vi "Main.vi"() -> ()   [LabVIEW 2018]
doc: "The myRIO Project template acquires acceleration data from the onboard accelerometer and displays the changes of acceleration values in a waveform chart."
uses:
  <vilib>/myRIO/Instrument Drivers/Utilities/Utilities.lvlib
  <vilib>/imath/engines/lvmath2/RunTimeEngine/Managers/WorkSpace/UID Generator.vi
  <vilib>/imath/engines/lvmath/Plug In/_Char/NIMS_CH_String to Character Array.vi
  <vilib>/imath/engines/lvmath/Plug In/_Char/NIMS_CH_character datatype.ctl
  <vilib>/imath/engines/lvmath2/RunTimeEngine/IndexRead/NIMS V(S).vi
  <vilib>/imathl/engines/lvmath/Functions/Error Handling/Create Error.vi
  <vilib>/imath/engines/lvmath2/RunTimeEngine/LocalVariableDefStatement/MC_LocalVariableDefStatement_Display.vi
  <vilib>/imath/engines/lvmath2/RunTimeEngine/RunTimeType/NIMS_RunTimeType_From StrictType (excl LVString).vi
  <vilib>/imath/engines/lvmath2/RunTimeEngine/Managers/SymbolTable/Clear UID.vi
  <vilib>/imath/engines/lvmath2/RunTimeEngine/Managers/SymbolTable/NIMS_WorkSpace.lvlib
  <vilib>/imath/engines/lvmath2/RunTimeEngine/NodeEndStatement/NIMS_NodeEndStatement_Output.vi
  <vilib>/imath/engines/lvmath2/RunTimeEngine/ErrorHandling/NIMS_Finalize Error.vi
  <vilib>/Analysis/NI_AALPro.lvlib
  <vilib>/imath/engines/lvmath2/RunTimeEngine/IndexReplace/NIMS M(S,S)=S.vi
  <vilib>/imath/engines/lvmath2/RunTimeEngine/ErrorHandling/NIMS_Create Error From Enums.vi
  <vilib>/imath/engines/lvmath2/RunTimeEngine/RangeToken/NIMS_Range_R2 - Integer.vi
  <vilib>/imath/engines/lvmath2/RunTimeEngine/CommandStatement/MC_CommandStatement_break.vi
  <vilib>/imath/engines/lvmath2/RunTimeEngine/IndexRead/NIMS M(S,S).vi
  <vilib>/robotics/Navigation/shared/WorldMap/OccupancyGridWorldMap/NI_Robotics_OccupancyGridWorldMap.lvclass
  <vilib>/imath/engines/lvmath2/RunTimeEngine/BuiltInFunctions/acos/NIMS_acos(C).vi
  <vilib>/Analysis/coordinate.llb/2D Cartesian Coordinate Rotation (Scalar).vi
  <vilib>/robotics/Navigation/shared/MapNode/OccupancyGridNode/NI_Robotics_OccupancyGridMapNode.lvclass
  C:/Program Files (x86)/National Instruments/LabVIEW 2018/vi.lib/robotics/Navigation/shared/MapNode/AbstractAstarNode/NI_Robotics_AbstractAstarNode.lvclass
  <vilib>/imath/engines/lvmath2/RunTimeEngine/BuiltInFunctions/round/NIMS_round(DBL-S).vi
  <vilib>/imath/engines/lvmath2/RunTimeEngine/BuiltInFunctions/char/NIMS_char.vi
  <vilib>/imath/engines/lvmath/Plug In/_Char/NIMS_CH_String CV to Character 2D.vi
  <vilib>/imath/engines/lvmath2/RunTimeSupport/NIMS_Error if Not Equal.vi
  <vilib>/imath/engines/lvmath2/RunTimeEngine/BuiltInFunctions/min/2 inputs/NIMS_min(RG,RG)-no size check.vi
  <vilib>/imath/engines/lvmath2/RunTimeEngine/BuiltInFunctions/max/2 inputs/NIMS_max(RG,RG)-no size check.vi
  <vilib>/imath/engines/lvmath/Plug In/_Char/NIMS_CH_Character 2D to String 1D.vi
  <vilib>/imath/engines/lvmath2/RunTimeEngine/BuiltInFunctions/mod/NIMS_mod_no_size_check.vi
  <vilib>/imath/engines/lvmath2/RunTimeEngine/VariableToken/NIMS_VariableToken_CondDefined.vi
  <vilib>/imath/engines/lvmath/Functions/Error Handling/MergeErrorsWrapper.vi
panel:
  out "field":i32[][](array[numeric])
  out "error out":errorcluster
  in  "stop":bool
  in  "Tab Control":enum32{"Main", "Settings"}(tab)
  out "Dist Finish":dbl
  out "Theta Finish":dbl
  out "Read Camera":bool
  out "Data":string
  out "Position":cluster{"X":dbl, "Y":dbl, "Theta":dbl}
  out "X Finish":string[](array[string])
  out "Y Finish":string[](array[string])
  out "G":i32[][](array[numeric])
  in  "Motor Controller ID#  (I2C Address)":u8=1 min=1 max=4
  in  "Motor Controller ID#  (I2C Address) 2":u8=2 min=1 max=4
  in  "Servo Controller ID#  (I2C Address) 3":u8=3 min=1 max=4
  in  "Controller myRIO MXP Port A/B":tag="A/I2C"
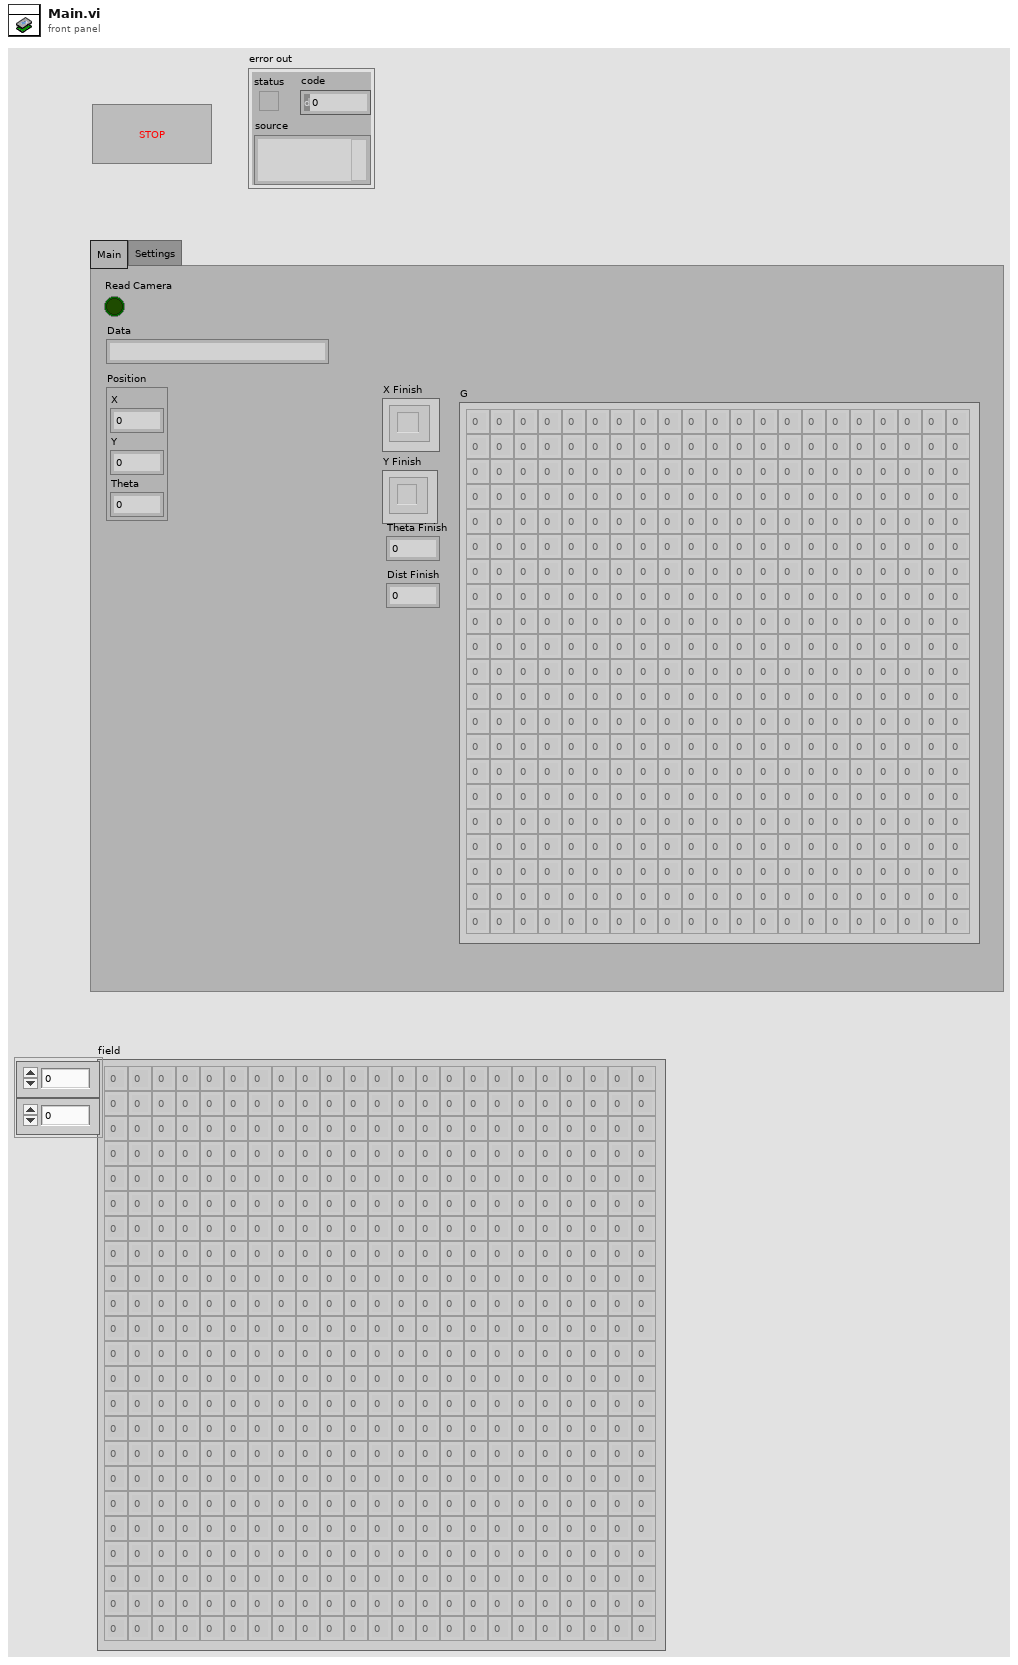
[diagram p1: front panel]
types:
  T1 = typedef "NIMS_CH_character datatype.ctl" = cluster{"Numeric":u8}
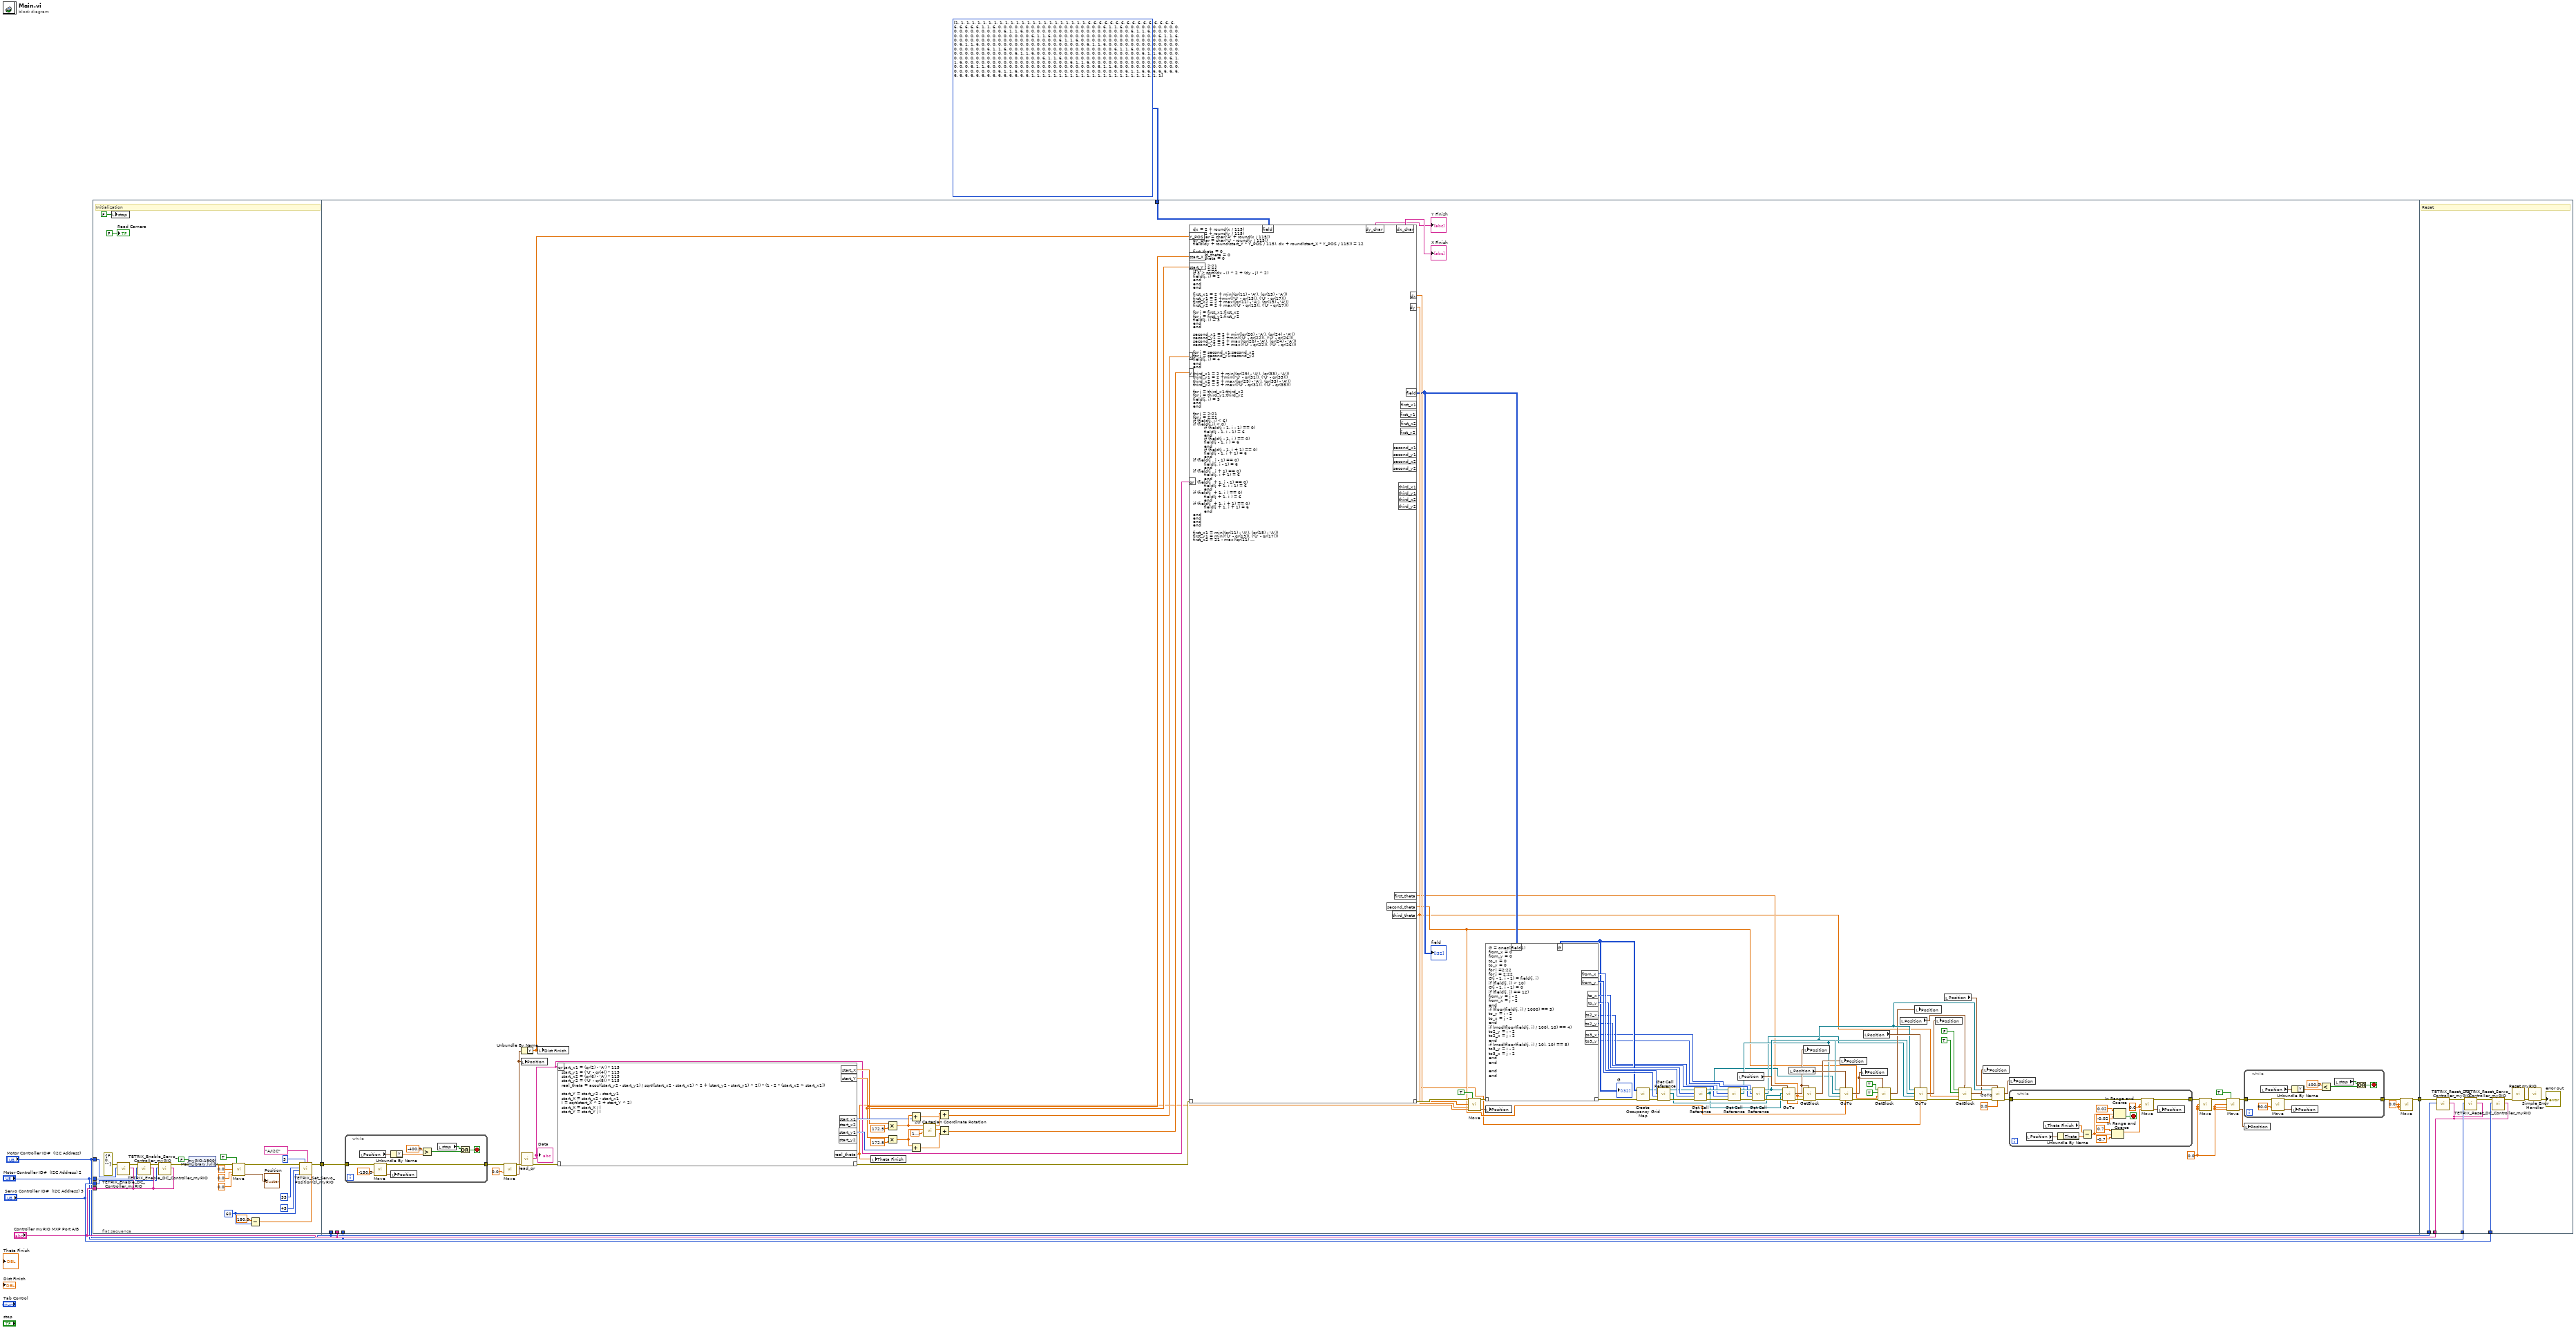
[diagram p0: block diagram]
diagram:
  n1 = flat-sequence {
    tunnel: "Motor Controller ID#  (I2C Address)" -> [w32]
    tunnel: "Motor Controller ID#  (I2C Address) 2" -> [w31]
    tunnel: "Controller myRIO MXP Port A/B" -> [w26]
    tunnel: "Servo Controller ID#  (I2C Address) 3" -> [w9]
    tunnel: [w10] -> w3
    tunnel: "Controller myRIO MXP Port A/B" -> [_]
    tunnel: "Motor Controller ID#  (I2C Address)" -> [_]
    tunnel: "Motor Controller ID#  (I2C Address) 2" -> [_]
    tunnel: w3 -> [w126]
    tunnel: u8[][] [[1, 1, 1, 1, 1, 1, 1, 1, 1, 1, 1, 1, 1, 1, 1, 1, 1, 1, 1, 1, 1, 1, 1], [1, 6, 6, 6, 6, 6, 6, 6, 6, 6, 6, 6, 6, 6, 6, 6, 6, 6, 6, 6, 6, 6, 1], [1, 6, 0, 0, 0, 0, 0, 0, 0, 0, 0, 0, 0, 0, 0, 0, 0, 0, 0, 0, 0, 6, 1], [1, 6, 0, 0, 0, 0, 0, 0, 0, 0, 0, 0, 0, 0, 0, 0, 0, 0, 0, 0, 0, 6, 1], [1, 6, 0, 0, 0, 0, 0, 0, 0, 0, 0, 0, 0, 0, 0, 0, 0, 0, 0, 0, 0, 6, 1], [1, 6, 0, 0, 0, 0, 0, 0, 0, 0, 0, 0, 0, 0, 0, 0, 0, 0, 0, 0, 0, 6, 1], [1, 6, 0, 0, 0, 0, 0, 0, 0, 0, 0, 0, 0, 0, 0, 0, 0, 0, 0, 0, 0, 6, 1], [1, 6, 0, 0, 0, 0, 0, 0, 0, 0, 0, 0, 0, 0, 0, 0, 0, 0, 0, 0, 0, 6, 1], [1, 6, 0, 0, 0, 0, 0, 0, 0, 0, 0, 0, 0, 0, 0, 0, 0, 0, 0, 0, 0, 6, 1], [1, 6, 0, 0, 0, 0, 0, 0, 0, 0, 0, 0, 0, 0, 0, 0, 0, 0, 0, 0, 0, 6, 1], [1, 6, 0, 0, 0, 0, 0, 0, 0, 0, 0, 0, 0, 0, 0, 0, 0, 0, 0, 0, 0, 6, 1], [1, 6, 0, 0, 0, 0, 0, 0, 0, 0, 0, 0, 0, 0, 0, 0, 0, 0, 0, 0, 0, 6, 1], [1, 6, 0, 0, 0, 0, 0, 0, 0, 0, 0, 0, 0, 0, 0, 0, 0, 0, 0, 0, 0, 6, 1], [1, 6, 0, 0, 0, 0, 0, 0, 0, 0, 0, 0, 0, 0, 0, 0, 0, 0, 0, 0, 0, 6, 1], [1, 6, 0, 0, 0, 0, 0, 0, 0, 0, 0, 0, 0, 0, 0, 0, 0, 0, 0, 0, 0, 6, 1], [1, 6, 0, 0, 0, 0, 0, 0, 0, 0, 0, 0, 0, 0, 0, 0, 0, 0, 0, 0, 0, 6, 1], [1, 6, 0, 0, 0, 0, 0, 0, 0, 0, 0, 0, 0, 0, 0, 0, 0, 0, 0, 0, 0, 6, 1], [1, 6, 0, 0, 0, 0, 0, 0, 0, 0, 0, 0, 0, 0, 0, 0, 0, 0, 0, 0, 0, 6, 1], [1, 6, 0, 0, 0, 0, 0, 0, 0, 0, 0, 0, 0, 0, 0, 0, 0, 0, 0, 0, 0, 6, 1], [1, 6, 0, 0, 0, 0, 0, 0, 0, 0, 0, 0, 0, 0, 0, 0, 0, 0, 0, 0, 0, 6, 1], [1, 6, 0, 0, 0, 0, 0, 0, 0, 0, 0, 0, 0, 0, 0, 0, 0, 0, 0, 0, 0, 6, 1], [1, 6, 6, 6, 6, 6, 6, 6, 6, 6, 6, 6, 6, 6, 6, 6, 6, 6, 6, 6, 6, 6, 1], [1, 1, 1, 1, 1, 1, 1, 1, 1, 1, 1, 1, 1, 1, 1, 1, 1, 1, 1, 1, 1, 1, 1]] ("Field") -> [w105]
    tunnel: [w59] -> w1
    tunnel: "Controller myRIO MXP Port A/B" -> [w4697]
    tunnel: "Motor Controller ID#  (I2C Address)" -> [w4701]
    tunnel: "Motor Controller ID#  (I2C Address) 2" -> [w4700]
    tunnel: "Servo Controller ID#  (I2C Address) 3" -> [w4698]
    tunnel: w1 -> [w4693]
    frame #0 {
      w16 = u8 60 ("Servo 4 Position (0 - 180 degrees)")
      # "Initialization"
      n2 = local write "stop"(FALSE ("Stop")) -> ()
      n3 = call <vilib>:"TETRIX_Enable_DC_Controller_myRIO.vi"("myRIO MXP Port A/B"=w26, "Controller ID#  (I2C Address)"=w32, "Error/Flow In"=errorcluster {"status"=FALSE, "code"=0, "source"=""}) -> ("Error/Flow Out"=w33:errorcluster)  [unwired: 4 in]
      n4 = call <vilib>:"TETRIX_Enable_DC_Controller_myRIO.vi"("myRIO MXP Port A/B"=w26, "Controller ID#  (I2C Address)"=w31, "Error/Flow In"=w33) -> ("Error/Flow Out"=w29:errorcluster)  [unwired: 4 in]
      n5 = call <vilib>:"TETRIX_Enable_Servo_Controller_myRIO.vi"("myRIO MXP Port A/B"=w26, "Controller ID#  (I2C Address)"=w9, "Error/Flow In"=w29) -> ("Error/Flow Out"=w28:errorcluster)  [unwired: 4 in]
      n6 = shared-variable "myRIO-1900\\MainLibrary.lvlib\\stop"(FALSE ("Stop"), error in=w28) -> (error out=w23:errorcluster)
      n7 = call "Move.vi"("Error/Flow In"=w23, "Reset"=TRUE, "x (mm/s)"=0.0, "y (mm/s)"=0.0, "theta (rad/s)"=0.0) -> ("Error/Flow Out"=w11:errorcluster, "Position"=→"Position":cluster{"X":dbl, "Y":dbl, "Theta":dbl})  [unwired: 9 in]
      n8 = Subtract(x=180.0, y=w16) -> (x-y=w15:dbl)
      n9 = call <vilib>:"TETRIX_Set_Servo_Position(s)_myRIO.vi"("Servo 4 Position (0 - 180 degrees)"=w15, "myRIO MXP Port A/B"=tag "A/I2C", "Controller ID#  (I2C Address)"=u8 3, "Servo 3 Position (0 - 180 degrees)"=w16, "Servo 2 Position (0 - 180 degrees)"=u8 45, "Servo 1 Position (0 - 180 degrees)"=u8 35 ("Controller ID#  (I2C Address)"), "Error/Flow In"=w11) -> ("Error/Flow Out"=w10:errorcluster)  [unwired: 2 in]
      "Read Camera" <- FALSE ("Read Camera")
    }
    frame #1 {
      w58 = 0.0 ("x (mm/s)")
      w63 = 0.0 ("x (mm/s)")
      n10 = while {
        tunnel: [w4688] -> w125
        tunnel: w126 -> [w4689]
        stop <- w4683 stop-if-true
        n11 = local read "Position"() -> (w4692:cluster{"X":dbl, "Y":dbl, "Theta":dbl})
        n12 = call "Move.vi"("Error/Flow In"=w4689, "y (mm/s)"=-150.0) -> ("Error/Flow Out"=w4688:errorcluster, "Position"=w4687:cluster{"X":dbl, "Y":dbl, "Theta":dbl})  [unwired: 12 in]
        n13 = Unbundle By Name(w4692) -> ("Y"=w4691:dbl)
        n14 = local write "Position"(w4687) -> ()
        n15 = Greater?(x=-400.0, y=w4691) -> (0:w4684:bool)
        n16 = local read "stop"() -> (w4685:bool)
        n17 = Or(x=w4685, y=w4684) -> (x .or. y?=w4683:bool)
      }
      n18 = call "Move.vi"("Error/Flow In"=w125, "y (mm/s)"=0.0) -> ("Error/Flow Out"=w127:errorcluster, "Position"=w106:cluster{"X":dbl, "Y":dbl, "Theta":dbl})  [unwired: 12 in]
      n19 = Unbundle By Name(w106) -> ("Y"=w89:dbl)
      n20 = local write "Position"(w106) -> ()
      n21 = call "read_qr.vi"("error in"=w127) -> ("error out"=w108:errorcluster, "Data"=w109:string)  [unwired: 8 in]
      "Data" <- w109
      n22 = local write "Dist Finish"(w89) -> ()
      n23 = mathscript code="start_x1 = (qr(2) - 'A') * 115\nstart_y1 = ('U' - qr(4)) * 115\nstart_x2 = (qr(6) - 'A') * 115\nstart_y2 = ('U' - qr(8)) * 115\nreal_theta = acos((start_y2 - start_y1) / sqrt((start_x2 - start_x1) ^ 2 + (start_y2 - start_y1) ^ 2)) * (1 - 2 * (start_x2 > start_x1))\n\nstart_Y = start_y2 - start_y1\nstart_X = start_x2 - start_x1\nl = sqrt(start_X ^ 2 + start_Y ^ 2)\nstart_X = start_X / l\nstart_Y = start_Y / l"("??"=w108, "qr"=w109) -> ("??"=w107:errorcluster, "real_theta"=w57:cdb, "start_x1"=w115:i32, "start_y1"=w114:i32, "start_X"=w113:dbl, "start_Y"=w112:dbl)  [unwired: 2 out]
      n24 = local write "Theta Finish"(w57) -> ()
      n25 = Multiply(x=w113, y=172.5) -> (x*y=w118:dbl)
      n26 = Multiply(x=w112, y=172.5) -> (x*y=w119:dbl)
      n27 = Add(x=w118, y=w115) -> (x+y=w120:dbl)
      n28 = Add(x=w119, y=w114) -> (x+y=w122:dbl)
      n29 = call-poly <vilib>:"2D Cartesian Coordinate Rotation.vi"("theta"=1.5707963267948966, "y"=w119, "x"=w118) -> ("y out"=w123:dbl, "x out"=w121:dbl)  [unwired: 6 in, 1 out]
      n30 = Add(x=w121, y=w120) -> (x+y=w111:dbl)
      n31 = Add(x=w123, y=w122) -> (x+y=w110:dbl)
      n32 = mathscript code="dx = 2 + round(x / 115)\ndy = 2 + round(y / 115)\ndx_char = char('A' + round(x / 115))\ndy_char = char('U' - round(y / 115))\nfield(dy + round(start_Y * Y_POS / 115), dx + round(start_X * Y_POS / 115)) = 12\n\nfirst_theta = 0\nsecond_theta = 0\nthird_theta = 0\n\nfor i = 2:21\nfor j = 2:21\nif 3 > sqrt((dx - i) ^ 2 + (dy - j) ^ 2)\nfield(j, i) = 2\nend\nend\nend\n\nfirst_x1 = 2 + min((qr(11) - 'A'), (qr(15) - 'A'))\nfirst_y1 = 2 +min(('U' - qr(13)), ('U' - qr(17)))\nfirst_x2 = 2 + max((qr(11) - 'A'), (qr(15) - 'A'))\nfirst_y2 = 2 + max(('U' - qr(13)), ('U' - qr(17)))\n\nfor i = first_x1:first_x2\nfor j = first_y1:first_y2\nfield(j, i) = 3\nend\nend\n\nsecond_x1 = 2 + min((qr(20) - 'A'), (qr(24) - 'A'))\nsecond_y1 = 2 +min(('U' - qr(22)), ('U' - qr(26)))\nsecond_x2 = 2 + max((qr(20) - 'A'), (qr(24) - 'A'))\nsecond_y2 = 2 + max(('U' - qr(22)), ('U' - qr(26)))\n\nfor i = second_x1:second_x2\nfor j = second_y1:second_y2\nfield(j, i) = 4\nend\nend\n\nthird_x1 = 2 + min((qr(29) - 'A'), (qr(33) - 'A'))\nthird_y1 = 2 +min(('U' - qr(31)), ('U' - qr(35)))\nthird_x2 = 2 + max((qr(29) - 'A'), (qr(33) - 'A'))\nthird_y2 = 2 + max(('U' - qr(31)), ('U' - qr(35)))\n\nfor i = third_x1:third_x2\nfor j = third_y1:third_y2\nfield(j, i) = 5\nend\nend\n\nfor i = 2:21\nfor j = 2:21\nif (field(j, i) < 6)\nif (field(j,i) > 0)\n        if (field(j - 1, i - 1) == 0)\n        field(j - 1, i - 1) = 6\n        end\n        if (field(j - 1, i ) == 0)\n        field(j - 1, i ) = 6\n        end\n        if (field(j - 1, i + 1) == 0)\n        field(j - 1, i + 1) = 6\n        end\nif (field(j , i - 1) == 0)\n        field(j, i - 1) = 6\n        end\nif (field(j , i + 1) == 0)\n        field(j, i + 1) = 6\n        end\nif (field(j  + 1, i - 1) == 0)\n        field(j + 1, i - 1) = 6\n        end\nif (field(j  + 1, i ) == 0)\n        field(j + 1, i ) = 6\n        end\nif (field(j  + 1, i + 1) == 0)\n        field(j + 1, i + 1) = 6\n        end\nend\nend\nend\nend\n\nfirst_x1 = min((qr(11) - 'A'), (qr(15) - 'A'))\nfirst_y1 = min(('U' - qr(13)), ('U' - qr(17)))\nfirst_x2 = 21 - max((qr(11) - 'A'), (qr(15) - 'A'))\nfirst_y2 = 21 - max(('U' - qr(13)), ('U' - qr(17)))\n\nmin_dist = min(first_x1, min(first_x2, min(first_y1, first_y2)))\nif min_dist == first_x1\n    field(2 + first_y1 + 1, 2 + 21 -first_x2 + 2) = 3000\n    first_theta = pi / 2\nend\nif min_dist == first_x2\n    field(2 + first_y1 + 1, 2 + first_x1 - 2) = 3000\n    first_theta = -pi / 2\nend\nif min_dist == first_y1\n    field(2 + 21 - first_y2 + 2, 2 + first_x1 + 1) = 3000\n    first_theta = pi\nend\nif min_dist == first_y2\n    field(2 + first_y1 - 2, 2 + first_x1 + 1) = 3000\n    first_theta = 0\nend\n\nfirst_x1 = min((qr(20) - 'A'), (qr(24) - 'A'))\nfirst_y1 = min(('U' - qr(22)), ('U' - qr(26)))\nfirst_x2 = 21 - max((qr(20) - 'A'), (qr(24) - 'A'))\nfirst_y2 = 21 - max(('U' - qr(22)), ('U' - qr(26)))\n\nmin_dist = min(first_x1, min(first_x2, min(first_y1, first_y2)))\nif min_dist == first_x1\n    field(2 + first_y1 + 1, 2 + 21 -first_x2 + 2) = field(2 + first_y1 + 1, 2 + 21 -first_x2 + 2) + 400\n    second_theta = pi / 2\nend\nif min_dist == first_x2\n    field(2 + first_y1 + 1, 2 + first_x1 - 2) = field(2 + first_y1 + 1, 2 + first_x1 - 2) + 400\n    second_theta = -pi / 2\nend\nif min_dist == first_y1\n    field(2 + 21 - first_y2 + 2, 2 + first_x1 + 1) =  field(2 + 21 - first_y2 + 2, 2 + first_x1 + 1) + 400\n    second_theta = pi\nend\nif min_dist == first_y2\n    field(2 + first_y1 - 2, 2 + first_x1 + 1) =  field(2 + first_y1 - 2, 2 + first_x1 + 1) + 400\n    second_theta = 0\nend\n\nfirst_x1 = min((qr(29) - 'A'), (qr(33) - 'A'))\nfirst_y1 = min(('U' - qr(31)), ('U' - qr(35)))\nfirst_x2 = 21 - max((qr(29) - 'A'), (qr(33) - 'A'))\nfirst_y2 = 21 - max(('U' - qr(31)), ('U' - qr(35)))\n\nmin_dist = min(first_x1, min(first_x2, min(first_y1, first_y2)))\nif min_dist == first_x1\n    field(2 + first_y1 + 1, 2 + 21 -first_x2 + 2) = field(2 + first_y1 + 1, 2 + 21 -first_x2 + 2) + 50\n    third_theta = pi / 2\nend\nif min_dist == first_x2\n    field(2 + first_y1 + 1, 2 + first_x1 - 2) = field(2 + first_y1 + 1, 2 + first_x1 - 2) + 50\n    third_theta = -pi / 2\nend\nif min_dist == first_y1\n    field(2 + 21 - first_y2 + 2, 2 + first_x1 + 1) =  field(2 + 21 - first_y2 + 2, 2 + first_x1 + 1) + 50\n    third_theta = pi\nend\nif min_dist == first_y2\n    field(2 + first_y1 - 2, 2 + first_x1 + 1) = field(2 + first_y1 - 2, 2 + first_x1 + 1) + 50\n    third_theta = 0\nend\n\ndx = dx - 2\ndy = dy - 2\ndx = (x + start_X * Y_POS)\ndy = (y + start_Y * Y_POS)\ndx_char = char('A' + round(dx / 115))\ndy_char = char('U' - round(dy / 115))"("??"=w107, "x"=w111, "y"=w110, "field"=w105, "qr"=w109, "start_X"=w113, "start_Y"=w112, "Y_POS"=w89) -> ("??"=w102:errorcluster, "dx"=w100:dbl, "dy"=w99:dbl, "field"=w91:i32[][], "dx_char"=→"X Finish":string[], "dy_char"=→"Y Finish":string[], "first_theta"=w34:dbl, "second_theta"=w38:dbl, "third_theta"=w37:dbl)  [unwired: 12 out]
      "field" <- w91
      n33 = call "Move.vi"("Error/Flow In"=w102, "Reset"=TRUE, "x (mm/s)"=w100, "y (mm/s)"=w99, "theta (rad/s)"=w57) -> ("Error/Flow Out"=w94:errorcluster, "Position"=w98:cluster{"X":dbl, "Y":dbl, "Theta":dbl})  [unwired: 9 in]
      n34 = mathscript code="G = ones(21, 21)\nfrom_x = 0\nfrom_y = 0\nto_x = 0\nto_y = 0\nfor i =2:22\nfor j = 2:22\nG(j - 1, i - 1) = field(j, i)\nif (field(j, i) > 10)\nG(j - 1, i - 1) = 0\nif (field(j, i) == 12)\nfrom_y = i - 2\nfrom_x = j - 2\nend\nif (floor(field(j, i) / 1000) == 3)\nto_y = i - 2\nto_x = j - 2\nend\nif (mod(floor(field(j, i) / 100), 10) == 4)\nto2_y = i - 2\nto2_x = j - 2\nend\nif (mod(floor(field(j, i) / 10), 10) == 5)\nto3_y = i - 2\nto3_x = j - 2\nend\nend\n\nend\nend"("??"=w94, "field"=w91) -> ("??"=w97:errorcluster, "from_x"=w96:i32, "from_y"=w95:i32, "to_x"=w93:i32, "to_y"=w92:i32, "to2_x"=w83:i32, "to2_y"=w82:i32, "to3_x"=w78:i32, "to3_y"=w77:i32, "G"=w90:i32[][])
      "G" <- w90
      n35 = local write "Position"(w98) -> ()
      n36 = call <vilib>:"Create Occupancy Grid Map.vi"("error in (no error)"=w97, "occupancy grid"=w90) -> ("error out"=w88:errorcluster, "map reference out"=w86:refnum<data-value>)  [unwired: 8 in]
      n37 = call <vilib>:"Get Cell Reference.vi"("error in (no error)"=w88, "y"=w95, "x"=w96, "map reference in"=w86) -> ("error out"=w87:errorcluster, "cell reference"=w36:refnum<data-value>, "map reference out"=w85:refnum<data-value>)  [unwired: 4 in, 1 out]
      n38 = call <vilib>:"Get Cell Reference.vi"("error in (no error)"=w87, "y"=w92, "x"=w93, "map reference in"=w85) -> ("error out"=w81:errorcluster, "cell reference"=w35:refnum<data-value>, "map reference out"=w84:refnum<data-value>)  [unwired: 4 in, 1 out]
      n39 = call <vilib>:"Get Cell Reference.vi"("error in (no error)"=w81, "y"=w82, "x"=w83, "map reference in"=w84) -> ("error out"=w79:errorcluster, "cell reference"=w40:refnum<data-value>, "map reference out"=w80:refnum<data-value>)  [unwired: 4 in, 1 out]
      n40 = local read "Position"() -> (w75:cluster{"X":dbl, "Y":dbl, "Theta":dbl})
      n41 = call <vilib>:"Get Cell Reference.vi"("error in (no error)"=w79, "y"=w77, "x"=w78, "map reference in"=w80) -> ("error out"=w76:errorcluster, "cell reference"=w39:refnum<data-value>, "map reference out"=w70:refnum<data-value>)  [unwired: 4 in, 1 out]
      n42 = call "GoTo.vi"("theta"=w34, "Position"=w75, "error in (no error)"=w76, "goal reference"=w35, "start reference"=w36, "map reference in"=w70) -> ("Error/Flow Out"=w56:errorcluster, "New Position"=w47:cluster{"X":dbl, "Y":dbl, "Theta":dbl})  [unwired: 4 in]
      n43 = local read "Position"() -> (w74:cluster{"X":dbl, "Y":dbl, "Theta":dbl})
      n44 = local write "Position"(w47) -> ()
      n45 = call "GetBlock.vi"("Position"=w47, "Error/Flow Out"=w56, "Theta"=w34) -> ("Error/Flow Out 2"=w48:errorcluster, "New Position"=w55:cluster{"X":dbl, "Y":dbl, "Theta":dbl})  [unwired: 7 in]
      n46 = local write "Position"(w55) -> ()
      n47 = call "GoTo.vi"("theta"=w38, "Position"=w74, "error in (no error)"=w48, "goal reference"=w40, "start reference"=w35, "map reference in"=w70) -> ("Error/Flow Out"=w54:errorcluster, "New Position"=w52:cluster{"X":dbl, "Y":dbl, "Theta":dbl})  [unwired: 4 in]
      n48 = local write "Position"(w52) -> ()
      n49 = local read "Position"() -> (w73:cluster{"X":dbl, "Y":dbl, "Theta":dbl})
      n50 = call "GetBlock.vi"("Position"=w52, "Error/Flow Out"=w54, "Theta"=w38, "Change"=TRUE, "Right Arm"=TRUE) -> ("Error/Flow Out 2"=w53:errorcluster, "New Position"=w51:cluster{"X":dbl, "Y":dbl, "Theta":dbl})  [unwired: 5 in]
      n51 = local read "Position"() -> (w44:cluster{"X":dbl, "Y":dbl, "Theta":dbl})
      n52 = local write "Position"(w51) -> ()
      n53 = call "GoTo.vi"("theta"=w37, "Position"=w73, "error in (no error)"=w53, "goal reference"=w39, "start reference"=w40, "map reference in"=w70) -> ("Error/Flow Out"=w46:errorcluster, "New Position"=w72:cluster{"X":dbl, "Y":dbl, "Theta":dbl})  [unwired: 4 in]
      n54 = local write "Position"(w72) -> ()
      n55 = local read "Position"() -> (w68:cluster{"X":dbl, "Y":dbl, "Theta":dbl})
      n56 = call "GetBlock.vi"("Position"=w44, "Error/Flow Out"=w46, "Theta"=w37, "Change"=TRUE, "Right Arm"=FALSE) -> ("Error/Flow Out 2"=w45:errorcluster, "New Position"=w43:cluster{"X":dbl, "Y":dbl, "Theta":dbl})  [unwired: 5 in]
      n57 = local write "Position"(w43) -> ()
      n58 = call "GoTo.vi"("theta"=0.0, "Position"=w68, "error in (no error)"=w45, "map reference in"=w70) -> ("Error/Flow Out"=w67:errorcluster, "New Position"=w71:cluster{"X":dbl, "Y":dbl, "Theta":dbl})  [unwired: 6 in]
      n59 = local write "Position"(w71) -> ()
      n60 = while {
        tunnel: w67 -> [w141]
        tunnel: [w139] -> w66
        stop <- w149 stop-if-true
        w142 = 0.0 ("x (mm/s)")
        n61 = local read "Position"() -> (w152:cluster{"X":dbl, "Y":dbl, "Theta":dbl})
        n62 = local read "Theta Finish"() -> (w150:dbl)
        n63 = Unbundle By Name(w152) -> ("Theta"=w151:dbl)
        n64 = Subtract(x=w150, y=w151) -> (x-y=w144:dbl)
        n65 = In Range and Coerce(upper limit=0.7, x=w144, lower limit=-0.7) -> (coerced(x)=w143:dbl)  [unwired: 1 out]
        n66 = In Range and Coerce(upper limit=0.02, x=w144, lower limit=-0.02) -> (In Range?=w149:bool)  [unwired: 1 out]
        n67 = call "Move.vi"("Error/Flow In"=w141, "x (mm/s)"=w142, "y (mm/s)"=w142, "theta (rad/s)"=w143) -> ("Error/Flow Out"=w139:errorcluster, "Position"=w140:cluster{"X":dbl, "Y":dbl, "Theta":dbl})  [unwired: 10 in]
        n68 = local write "Position"(w140) -> ()
      }
      n69 = call "Move.vi"("Error/Flow In"=w66, "x (mm/s)"=w63, "y (mm/s)"=w63, "theta (rad/s)"=w63) -> ("Error/Flow Out"=w65:errorcluster)  [unwired: 10 in, 1 out]
      n70 = call "Move.vi"("Error/Flow In"=w65, "Reset"=TRUE, "x (mm/s)"=w63, "y (mm/s)"=w63, "theta (rad/s)"=w63) -> ("Error/Flow Out"=w62:errorcluster, "Position"=w61:cluster{"X":dbl, "Y":dbl, "Theta":dbl})  [unwired: 9 in]
      n71 = while {
        tunnel: [w135] -> w60
        tunnel: w62 -> [w129]
        stop <- w130 stop-if-true
        n72 = local read "Position"() -> (w138:cluster{"X":dbl, "Y":dbl, "Theta":dbl})
        n73 = call "Move.vi"("Error/Flow In"=w129, "y (mm/s)"=50.0) -> ("Error/Flow Out"=w135:errorcluster, "Position"=w134:cluster{"X":dbl, "Y":dbl, "Theta":dbl})  [unwired: 12 in]
        n74 = Unbundle By Name(w138) -> ("Y"=w137:dbl)
        n75 = local write "Position"(w134) -> ()
        n76 = Less?(x=400.0, y=w137) -> (x < y?=w131:bool)
        n77 = local read "stop"() -> (w132:bool)
        n78 = Or(x=w132, y=w131) -> (x .or. y?=w130:bool)
      }
      n79 = local write "Position"(w61) -> ()
      n80 = call "Move.vi"("Error/Flow In"=w60, "x (mm/s)"=w58, "y (mm/s)"=w58, "theta (rad/s)"=w58) -> ("Error/Flow Out"=w59:errorcluster)  [unwired: 10 in, 1 out]
    }
    frame #2 {
      # "Reset"
      n81 = call <vilib>:"TETRIX_Reset_DC_Controller_myRIO.vi"("myRIO MXP Port A/B"=w4697, "Controller ID#  (I2C Address)"=w4701, "Error/Flow In"=w4693) -> ("Error/Flow Out"=w4702:errorcluster)  [unwired: 4 in]
      n82 = call <vilib>:"TETRIX_Reset_DC_Controller_myRIO.vi"("myRIO MXP Port A/B"=w4697, "Controller ID#  (I2C Address)"=w4700, "Error/Flow In"=w4702) -> ("Error/Flow Out"=w4699:errorcluster)  [unwired: 4 in]
      n83 = call <vilib>:"TETRIX_Reset_Servo_Controller_myRIO.vi"("myRIO MXP Port A/B"=w4697, "Controller ID#  (I2C Address)"=w4698, "Error/Flow In"=w4699) -> ("Error/Flow Out"=w4696:errorcluster)  [unwired: 4 in]
      n84 = call <vilib>:"Reset myRIO.vi"("error in (no error)"=w4696) -> ("error out"=w4695:errorcluster)  [unwired: 10 in]
      n85 = call <vilib>:"Simple Error Handler.vi"("error in (no error)"=w4695) -> ("error out"=→"error out":errorcluster)  [unwired: 4 in, 4 out]
    }
  }
